vi "Get Multiple Channels.vi"(9 "Channel names":string[](array[string]), 10 "Gateway IP Address (\"\": localhost)":string) -> (0 "error out":errorcluster, 1 "Channel.Units":string[](array[string]), 2 "Channel names out":string[](array[string]), 3 "Channel.Values":dbl[](array[numeric]))   [LabVIEW 2015, in "Set Channels.lvlib"]
uses:
  Set Channels.lvlib
  <vilib>/NI Veristand/Execution/Workspace/NI VeriStand - Get Multiple Channel Values.vi
  <vilib>/NI Veristand/Execution/Workspace/NI_VS Workspace ExecutionAPI.lvlib
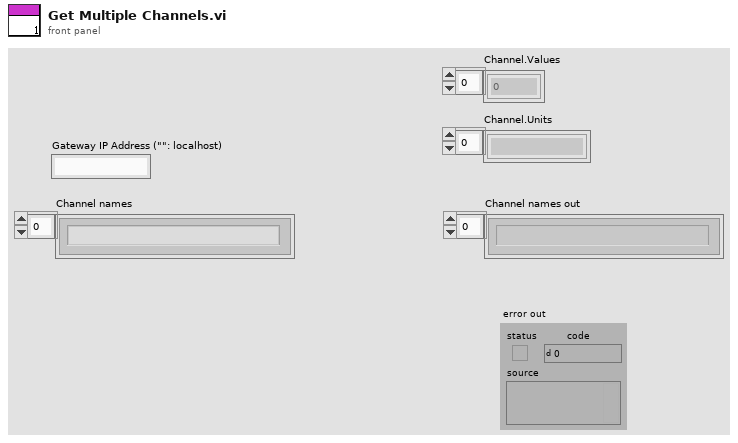
[diagram p1: front panel]
types:
  T1 = typedef "NI_VS Workspace ExecutionAPI.lvlib/WorkspaceAPI.ctl" = refnum<k24>
  T2 = typedef "NI_VS Workspace ExecutionAPI.lvlib/NodeInfo.ctl" = cluster{"Name":string, "FullPath":string, "Type":string, "IsChannel":bool, "Channel":cluster{"Unit":string, "Readable":bool, "Writable":bool, "Faultable":bool, "Scalable":bool, "RowDim":u32, "ColumnDim":u32, "Value Table Names":string[], "Value Table Values":dbl[]}, "IsWaveform":bool, "Waveform":cluster{"DataType":T3}}
  T3 = typedef "NI_VS Workspace ExecutionAPI.lvlib/Waveform Data Type.ctl" = enum16{"Double", "ComplexDouble"}
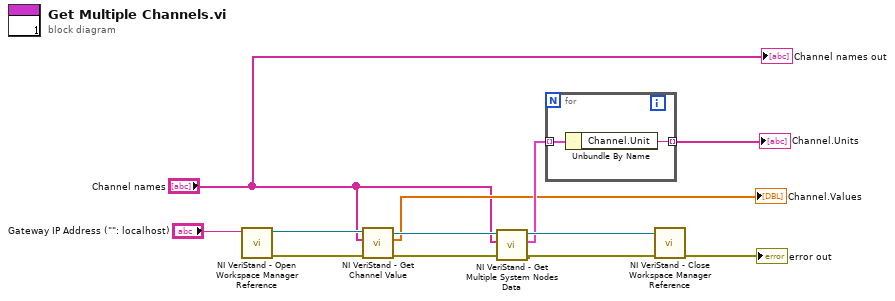
[diagram p0: block diagram]
diagram:
  n1 = call <vilib>:"NI VeriStand - Open Workspace Manager Reference.vi"("Gateway IP Address (\"\": localhost)"="Gateway IP Address (\"\": localhost)") -> ("error out"=w9:errorcluster, "WorkspaceManager"=w10:T1)  [unwired: 9 in]
  n2 = call-poly <vilib>:"NI VeriStand - Get Channel Value.vi"("error in (no error)"=w9, "Channels"="Channel names", "WorkspaceManager in"=w10) -> ("error out"=w8:errorcluster, "Values"=→"Channel.Values":dbl[], "WorkspaceManager out"=w7:T1)  [unwired: 6 in]
  n3 = call <vilib>:"NI VeriStand - Get Multiple System Nodes Data.vi"("error in (no error)"=w8, "Node Paths"="Channel names", "WorkspaceManager in"=w7) -> ("error out"=→"error out":errorcluster, "Nodes Data"=w4:T2[], "WorkspaceManager out"=w6:T1)  [unwired: 6 in]
  n4 = for {
    tunnel: w4 -> [w13] mode=indexing
    tunnel: [w12] -> w3 mode=indexing
    n5 = Unbundle By Name(w13) -> ("Channel.Unit"=w12:string)
  }
  "Channel.Units" <- w3
  n6 = call <vilib>:"NI VeriStand - Close Workspace Manager Reference.vi"("WorkspaceManager"=w6) -> ()  [unwired: 10 in, 1 out]
  "Channel names out" <- "Channel names"
